vi "Multiple DBL Key to 1D DBL Araray.vi"(7 "Section In":string, 8 "Error In":errorcluster, 10 "Keys In":string[](array[string]), 11 "Ref In":T1) -> (0 "Error Out":errorcluster, 2 "1D DBL Array Out":dbl[](array[numeric]) format="%#_f", 3 "Ref Out":T1)   [LabVIEW 2024]
uses:
  <vilib>/Utility/config.llb/Config Data RefNum.ctl
  <vilib>/Utility/config.llb/Read Key (Double).vi
  <vilib>/Utility/config.llb/NI_LVConfig.lvlib
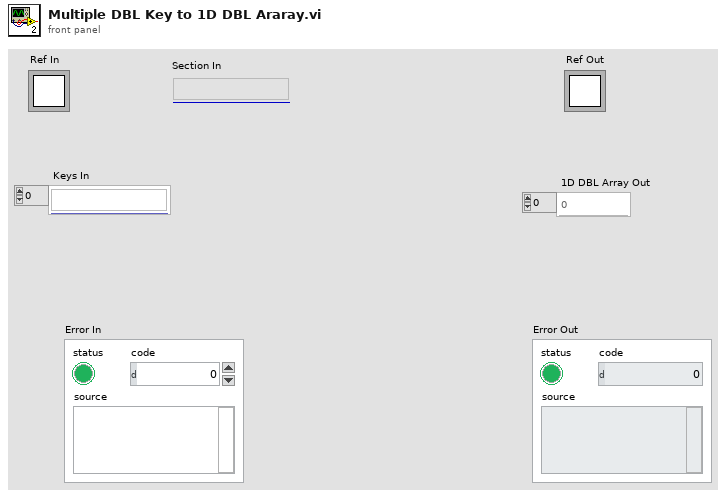
[diagram p1: front panel]
types:
  T1 = typedef "NI_LVConfig.lvlib/Config Data RefNum.ctl" = refnum<k1>
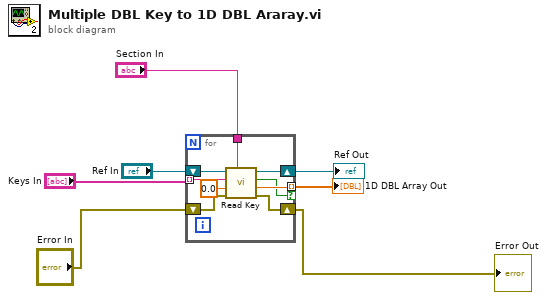
[diagram p0: block diagram]
diagram:
  n1 = for {
    shift-right: [w15] -> w5
    shift-left: "Ref In" -> [w16]
    tunnel: [w14] -> w1 mode=indexing if=w8
    tunnel: "Keys In" -> [w13] mode=indexing
    tunnel: "Section In" -> [w12]
    shift-right: [w9] -> w2
    shift-left: "Error In" -> [w10]
    n2 = call-poly <vilib>:"Read Key.vi"("section"=w12, "error in (no error)"=w10, "default value"=0.0, "key"=w13, "refnum"=w16) -> ("error out"=w9:errorcluster, "value"=w14:dbl, "found?"=w8:bool, "refnum out"=w15:T1)  [unwired: 3 in]
  }
  "Ref Out" <- w5
  "1D DBL Array Out" <- w1
  "Error Out" <- w2
